vi "Item.vi"(8 "error in (no error)":errorcluster, 10 "Key":string, 11 "StringMap in":refnum<class "StringMap.lvclass">) -> (0 "error out":errorcluster, 1 "Value":string, 3 "StringMap out":refnum<class "StringMap.lvclass">)   [LabVIEW 2013, in "LapDog.Collections.v1.Maps.lvlib" / "StringMap.lvclass"]
doc: "Returns a copy of the value associated with the given key.\n\nIf the key does not exist, error 510203 is returned."
uses:
  StringMap.lvclass
  StringMap.lvclass/StringMap.ctl
  LapDog.Collections.Common/String/String.lvclass
  ObjectMap/ObjectMap.lvclass
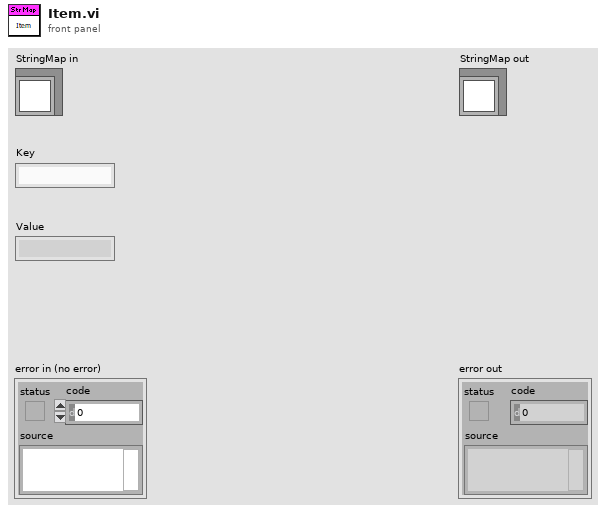
[diagram p1: front panel]
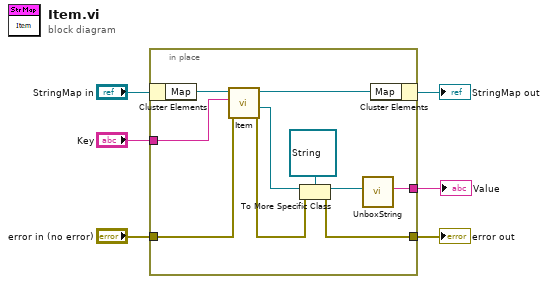
[diagram p0: block diagram]
diagram:
  n1 = in-place {
    in-place-border: "Key" -> [w14]
    in-place-border: "error in (no error)" -> [w13]
    in-place-border: [w7] -> w2
    in-place-border: [w11] -> w1
    n2 = in-place-cluster #1("StringMap in") -> ("Map"=w16:refnum<class "ObjectMap.lvclass">)
    n3 = call-dynamic "Item.vi"("error in (no error)"=w13, "Key"=w14, "Map in"=w16) -> ("error out"=w8:errorcluster, "Value"=w12:refnum<class>, "Map out"=w15:refnum<class "ObjectMap.lvclass">)  [unwired: 6 in]
    n4 = To More Specific Class(target class=refnum<class "String.lvclass"> refnum ("LapDog.Collections.v0.Common.lvlib:String.lvclass"), reference=w12, error in=w8) -> (specific class reference=w10:refnum<class "String.lvclass">, error out=w7:errorcluster)
    n5 = call "UnboxString.vi"("String in"=w10) -> ("String"=w11:string)  [unwired: 10 in]
    n6 = in-place-cluster #1("Map"=w15) -> (→"StringMap out":refnum<class "StringMap.lvclass">)
  }
  "error out" <- w2
  "Value" <- w1
